vi "Код команды (SubVI).vi"(11 "Команда управления":T1(ring)) -> (3 "Код команды":bool[](array[boolean]))   [LabVIEW 2015]
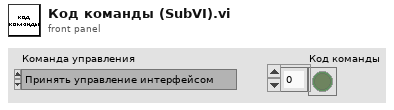
[diagram p1: front panel]
types:
  T1 = enum16{"Принять управление интерфейсом", "Синхронизация", "Передать ОС", "Начать самоконтроль ОУ", "Блокировать передатчик", "Разблокировать передатчик", "Блокировать признак неисправности ОУ", "Разблокировать признак неисправнотси ОУ", "Установить ОУ в исходное состояние", "Резерв", "Передать векорное слово", "Синхронизвция с СД", "Передать последнюю команду", "Передать слово ВСК ОУ", "Блокировать i-й передатчик", "Разблокировать i-й передатчик", "Резерв 2"}
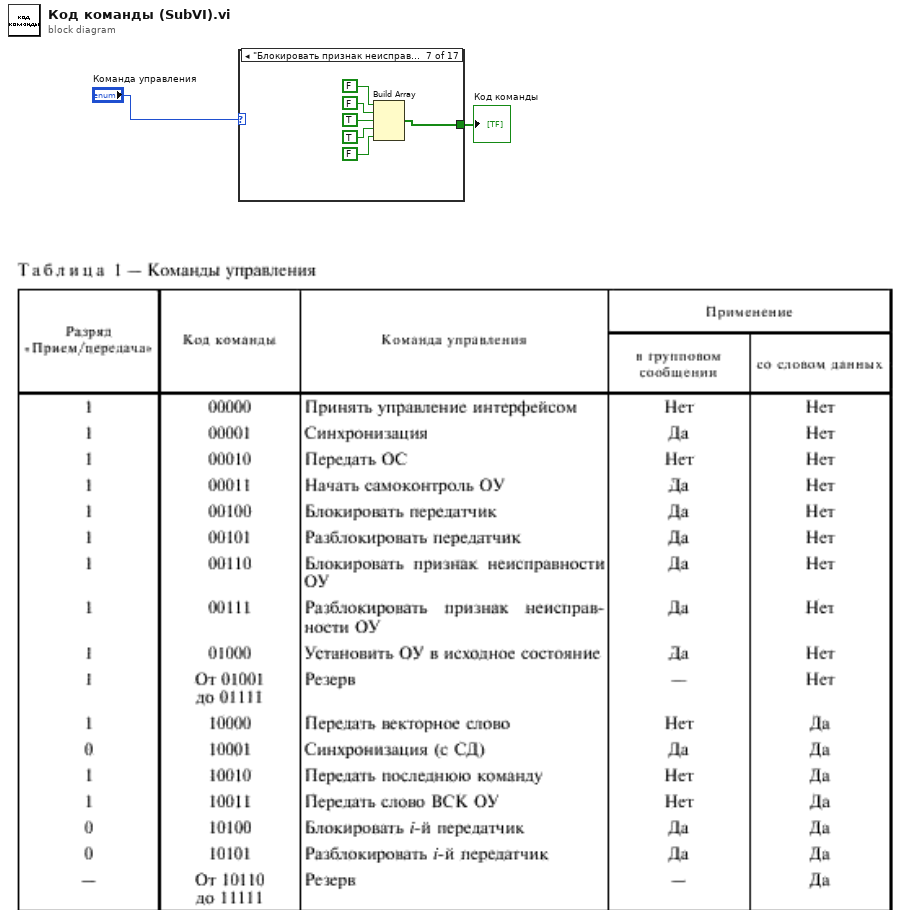
[diagram p0: block diagram]
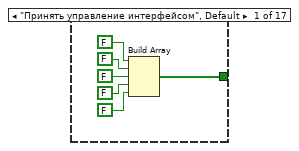
[diagram p2: hidden frame]
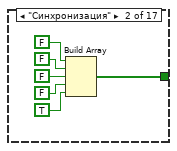
[diagram p3: hidden frame]
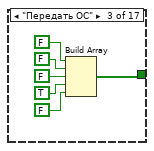
[diagram p4: hidden frame]
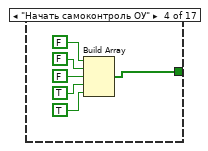
[diagram p5: hidden frame]
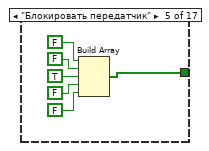
[diagram p6: hidden frame]
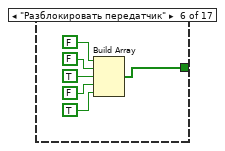
[diagram p7: hidden frame]
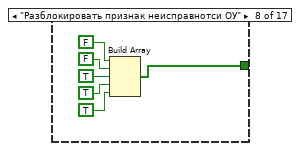
[diagram p8: hidden frame]
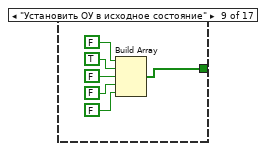
[diagram p9: hidden frame]
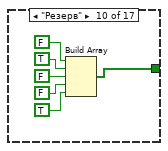
[diagram p10: hidden frame]
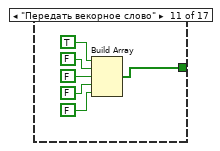
[diagram p11: hidden frame]
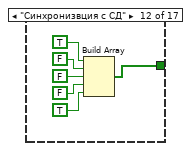
[diagram p12: hidden frame]
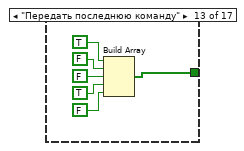
[diagram p13: hidden frame]
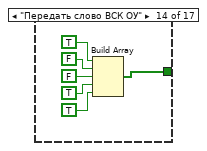
[diagram p14: hidden frame]
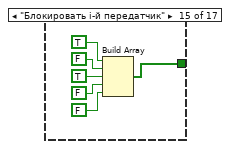
[diagram p15: hidden frame]
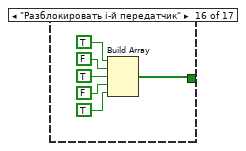
[diagram p16: hidden frame]
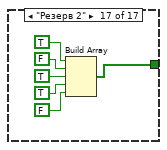
[diagram p17: hidden frame]
diagram:
  n1 = case shown="\"Блокировать признак неисправности ОУ\"" "Команда управления" {
    tunnel: [w3 w9 w15 w21 w27 w33 w39 w45 w51 w57 w63 w69 w75 w81 w87 w93 w99] -> w2
    frame "Принять управление интерфейсом", Default {
      n2 = Build Array(FALSE, FALSE, FALSE, FALSE, FALSE) -> (w3:bool[])
    }
    frame "Синхронизация" {
      n3 = Build Array(FALSE, FALSE, FALSE, FALSE, TRUE) -> (w9:bool[])
    }
    frame "Передать ОС" {
      n4 = Build Array(FALSE, FALSE, FALSE, TRUE, FALSE) -> (w15:bool[])
    }
    frame "Начать самоконтроль ОУ" {
      n5 = Build Array(FALSE, FALSE, FALSE, TRUE, TRUE) -> (w21:bool[])
    }
    frame "Блокировать передатчик" {
      n6 = Build Array(FALSE, FALSE, TRUE, FALSE, FALSE) -> (w27:bool[])
    }
    frame "Разблокировать передатчик" {
      n7 = Build Array(FALSE, FALSE, TRUE, FALSE, TRUE) -> (w33:bool[])
    }
    frame "Блокировать признак неисправности ОУ" {
      n8 = Build Array(FALSE, FALSE, TRUE, TRUE, FALSE) -> (w39:bool[])
    }
    frame "Разблокировать признак неисправнотси ОУ" {
      n9 = Build Array(FALSE, FALSE, TRUE, TRUE, TRUE) -> (w45:bool[])
    }
    frame "Установить ОУ в исходное состояние" {
      n10 = Build Array(FALSE, TRUE, FALSE, FALSE, FALSE) -> (w51:bool[])
    }
    frame "Резерв" {
      n11 = Build Array(FALSE, TRUE, FALSE, FALSE, TRUE) -> (w57:bool[])
    }
    frame "Передать векорное слово" {
      n12 = Build Array(TRUE, FALSE, FALSE, FALSE, FALSE) -> (w63:bool[])
    }
    frame "Синхронизвция с СД" {
      n13 = Build Array(TRUE, FALSE, FALSE, FALSE, TRUE) -> (w69:bool[])
    }
    frame "Передать последнюю команду" {
      n14 = Build Array(TRUE, FALSE, FALSE, TRUE, FALSE) -> (w75:bool[])
    }
    frame "Передать слово ВСК ОУ" {
      n15 = Build Array(TRUE, FALSE, FALSE, TRUE, TRUE) -> (w81:bool[])
    }
    frame "Блокировать i-й передатчик" {
      n16 = Build Array(TRUE, FALSE, TRUE, FALSE, FALSE) -> (w87:bool[])
    }
    frame "Разблокировать i-й передатчик" {
      n17 = Build Array(TRUE, FALSE, TRUE, FALSE, TRUE) -> (w93:bool[])
    }
    frame "Резерв 2" {
      n18 = Build Array(TRUE, FALSE, TRUE, TRUE, FALSE) -> (w99:bool[])
    }
  }
  "Код команды" <- w2
